vi "Knob Fill.vi"(9 "Default Value":dbl, 10 "Value":dbl, 11 "Knob Ref":refnum<vi>) -> ()   [LabVIEW 2019, in "User Interface.lvlib"]
doc: "Determines whether the knob fill type to use is one-way (min->max) or two way (default->min or default->max), and updates knob fill accordingly."
uses:
  User Interface.lvlib
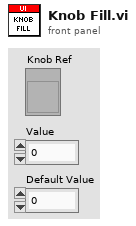
[diagram p1: front panel]
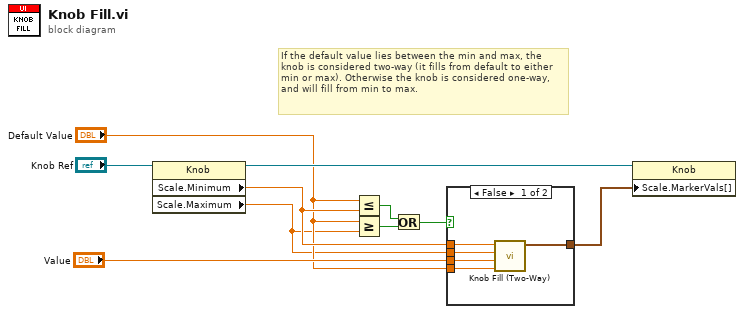
[diagram p0: block diagram]
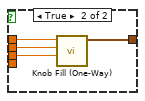
[diagram p2: hidden frame]
diagram:
  # "If the default value lies between the min and max, the knob is considered two-way (it fills from default to either min or max). Otherwise the knob is considered one-way, and will fill from min to max."
  n1 = property on="Property Node" class="Knob"(reference="Knob Ref") -> (reference out=w9:refnum<vi>, "Scale.Minimum"=w8:dbl, "Scale.Maximum"=w5:dbl)  [unwired: 1 in, 1 out]
  n2 = Less Or Equal?(x="Default Value", y=w8) -> (x <= y?=w3:bool)
  n3 = Greater Or Equal?(x="Default Value", y=w5) -> (x >= y?=w4:bool)
  n4 = Or(x=w3, y=w4) -> (x .or. y?=w2:bool)
  n5 = case shown="False" w2 {
    tunnel: w5 -> [w14 w19]
    tunnel: w8 -> [w15 w18]
    tunnel: "Value" -> [w13 w17]
    tunnel: "Default Value" -> [w12 _]
    tunnel: [w11 w16] -> w1
    frame False {
      n6 = call "Knob Fill (Two-Way).vi"("Default Value"=w12, "Value"=w13, "Maximum"=w14, "Minimum"=w15) -> ("Marker Values"=w11:cluster{"Value":dbl, "Color Box":u32}[])  [unwired: 7 in]
    }
    frame True {
      n7 = call "Knob Fill (One-Way).vi"("Value"=w17, "Maximum"=w19, "Minimum"=w18) -> ("Marker Values"=w16:cluster{"Value":dbl, "Color Box":u32}[])  [unwired: 8 in]
    }
  }
  n8 = property on="Property Node" class="Knob"(reference=w9, "Scale.MarkerVals[]"=w1) -> ()  [unwired: 1 in, 2 out]
